vi "2D in 2D ersetzen.vi"(8 "error in (no error)":errorcluster caption="Fehler (Eingang, kein Fehler)", 9 "Teilarray":string[][](array[string]), 10 "Zeile":i32, 11 "Eingangs Array":string[][](array[string])) -> (0 "error out":errorcluster caption="Fehler (Ausgang)", 3 "Ausgangs Array":string[][](array[string]))   [LabVIEW 2020, in "EPA 1065.lvlib" / "Gas Analyzer Drift 1065-550.lvlib"]
uses:
  Gas Analyzer Drift 1065-550.lvlib
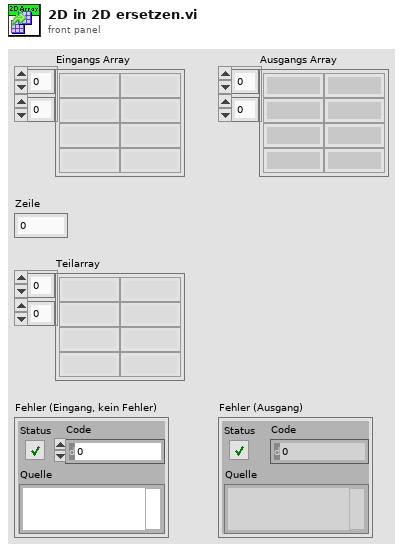
[diagram p1: front panel]
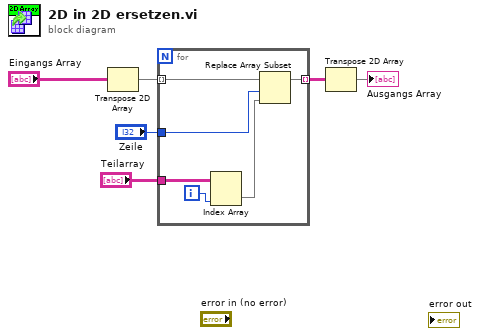
[diagram p0: block diagram]
diagram:
  n1 = Transpose 2D Array(2D array="Eingangs Array") -> (transposed array=w5:string[][])
  n2 = for {
    tunnel: w5 -> [w12] mode=indexing
    tunnel: "Teilarray" -> [w9]
    tunnel: "Zeile" -> [w11]
    tunnel: [w10] -> w4 mode=indexing
    i -> [w7]
    n3 = Index Array(array=w9, index (col)=w7) -> (element=w8:string[])  [unwired: 1 in]
    n4 = Replace Array Subset(array=w12, new element=w8, index=w11) -> (w10:string[])
  }
  n5 = Transpose 2D Array(2D array=w4) -> (transposed array=→"Ausgangs Array":string[][])
